vi "MPExxx_set_volt_curr.vi"(2 "error in (no error)":errorcluster, 3 "Set Current":dbl format="%.2f", 4 "Set Voltage":dbl format="%.2f", 5 "VISA session":refnum<visa-resource-name>) -> (0 "error out":errorcluster, 1 "dup VISA session":refnum<visa-resource-name>)   [LabVIEW 2015]
doc: "This VI form sets the voltage and current set points."
panel:
  # "MAGNA-POWER"
  # "Electronics"
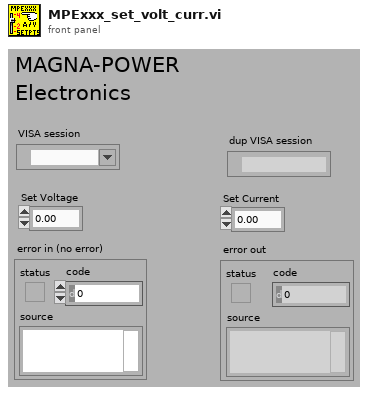
[diagram p1: front panel]
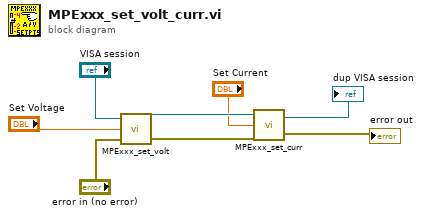
[diagram p0: block diagram]
diagram:
  n1 = call "MPExxx_set_volt.vi"("error in (no error)"="error in (no error)", "Set Voltage"="Set Voltage", "VISA session"="VISA session") -> ("error out"=w8:errorcluster, "dup VISA session"=w7:refnum<visa-resource-name>)
  n2 = call "MPExxx_set_curr.vi"("error in (no error)"=w8, "Set Current"="Set Current", "VISA session"=w7) -> ("error out"=→"error out":errorcluster, "dup VISA session"=→"dup VISA session":refnum<visa-resource-name>)
